vi "Glimpse delete acquisition directories.vi"(7 "error in":errorcluster) -> (3 "error out":errorcluster)   [LabVIEW 2011]
uses:
  GLIMPSE Globals.vi
panel:
  out "path":path
  out "String":string
  out "being deleted....":path
  in  "Cancel Button":bool
  in  "OK Button":bool
  out "Directories to be deleted":path[](array[path])
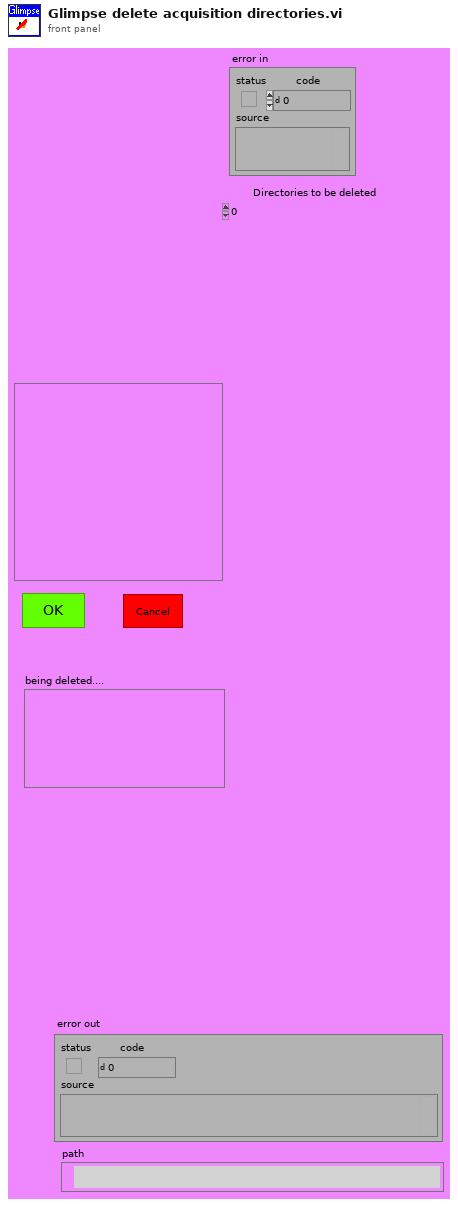
[diagram p1: front panel]
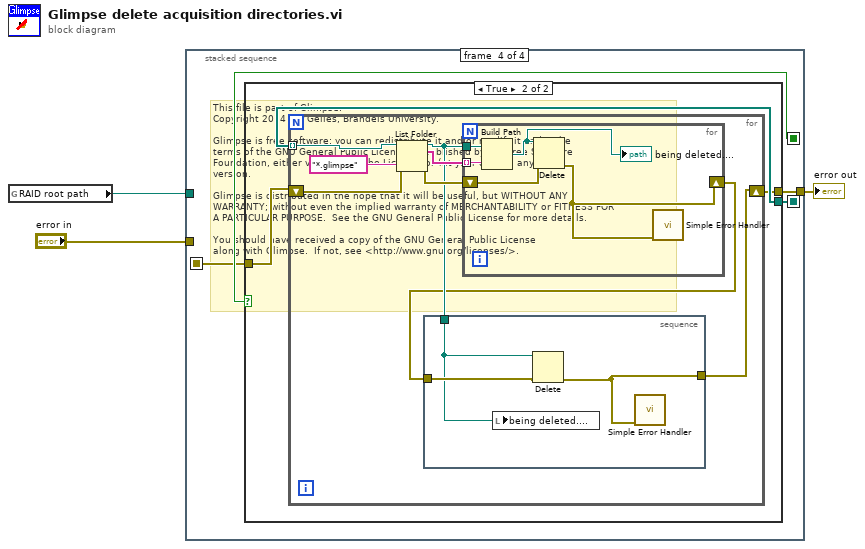
[diagram p0: block diagram]
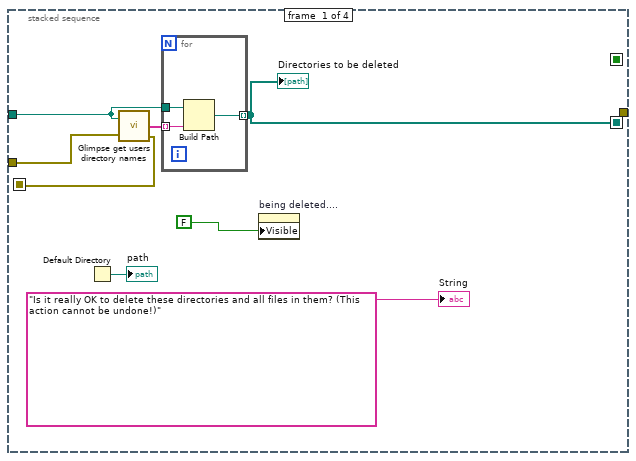
[diagram p2: hidden frame]
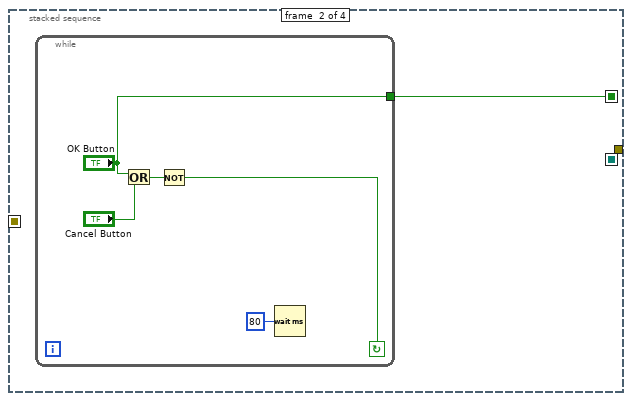
[diagram p3: hidden frame]
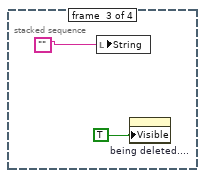
[diagram p4: hidden frame]
diagram:
  # "This file is part of Glimpse. \nCopyright 2014 Jeff Gelles, Brandeis University.    \n\nGlimpse is free software: you can redistribute it and/or modify it under the \nterms of the GNU General Public License as published by the Free Software \nFoundation, either version 3 of the License, or (at your option) any later \nversion.\n\nGlimpse is distributed in the hope that it will be useful, but WITHOUT ANY \nWARRANTY; without even the implied warranty of MERCHANTABILITY or FITNESS FOR \nA PARTICULAR PURPOSE.  See the GNU General Public License for more details.\n\nYou should have received a copy of the GNU General Public License\nalong with Glimpse.  If not, see <http://www.gnu.org/licenses/>."
  n1 = global read "GLIMPSE Globals.vi" "RAID root path"() -> (w2:path)
  n2 = stacked-sequence {
    seq-local: [w8 _ _ _] -> [_ _ _ w25]
    seq-local: [_ w15 _ _] -> [_ _ _ w26]
    seq-local: [w7 _ _ _] -> [_ _ _ w24]
    tunnel: "error in" -> [w11 _ _ _]
    tunnel: w2 -> [w9 _ _ _]
    tunnel: [_ _ _ w23] -> w1
    frame #0 {
      n3 = Default Directory() -> (→"path":path)
      n4 = call "Glimpse get users directory names.vi"("RAID root path"=w9, "error in"=w11) -> ("directory names"=w10:string[], "error out"=w7:errorcluster)  [unwired: 1 out]
      n5 = for {
        tunnel: w10 -> [w14] mode=indexing
        tunnel: w9 -> [w13]
        tunnel: [w12] -> w8 mode=indexing
        n6 = Build Path(base path=w13, name or relative path=w14) -> (appended path=w12:path)
      }
      "Directories to be deleted" <- w8
      n7 = property on="being deleted...." class="Path"("Visible"=FALSE) -> ()  [unwired: 2 in, 2 out]
      "String" <- "Is it really OK to delete these directories and all files in them? (This action cannot be undone!)" ("String")
    }
    frame #1 {
      n8 = while {
        tunnel: ["OK Button"] -> w15
        stop <- w17 continue-if-true
        n9 = Or(x="OK Button", y="Cancel Button") -> (x .or. y?=w19:bool)
        n10 = Not(x=w19) -> (.not. x?=w17:bool)
        n11 = Wait (ms)(milliseconds to wait=u32 80) -> ()  [unwired: 1 out]
      }
    }
    frame #2 {
      n12 = local write "String"("") -> ()
      n13 = property on="being deleted...." class="Path"("Visible"=TRUE) -> ()  [unwired: 2 in, 2 out]
    }
    frame #3 {
      n14 = case shown="True" w26 {
        tunnel: w25 -> [_ w30]
        tunnel: w24 -> [w27 w29]
        tunnel: [w27 w28] -> w23
        frame False {
        }
        frame True {
          n15 = for {
            tunnel: w30 -> [w38] mode=indexing
            shift-right: [w31] -> w28
            shift-left: w29 -> [w36]
            n16 = List Folder(path=w38, pattern="*.glimpse" ("name or relative path"), error in=w36) -> (path out=w33:path, filenames=w35:string[], error out=w34:errorcluster)  [unwired: 2 out]
            n17 = for {
              tunnel: w33 -> [w46]
              tunnel: w35 -> [w45] mode=indexing
              shift-right: [w42] -> w32
              shift-left: w34 -> [w44]
              n18 = Build Path(base path=w46, name or relative path=w45) -> (appended path=w43:path)
              "being deleted...." <- w43
              n19 = Delete(path (use dialog)=w43, error in=w44) -> (error out=w42:errorcluster)  [unwired: 5 out]
              n20 = call <vilib>:"Simple Error Handler.vi"("error in (no error)"=w42) -> ()  [unwired: 1 in, 8 out]
            }
            n21 = stacked-sequence {
              tunnel: w33 -> [w40]
              tunnel: w32 -> [w41]
              tunnel: [w39] -> w31
              frame #0 {
                n22 = local write "being deleted...."(w40) -> ()
                n23 = Delete(path (use dialog)=w40, error in=w41) -> (error out=w39:errorcluster)  [unwired: 5 out]
                n24 = call <vilib>:"Simple Error Handler.vi"("error in (no error)"=w39) -> ()  [unwired: 1 in, 8 out]
              }
            }
          }
        }
      }
    }
  }
  "error out" <- w1
